vi "global_vi.vi"() -> ()   [LabVIEW 2020]
panel:
  out "A":dbl
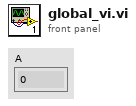
[diagram p1: front panel]
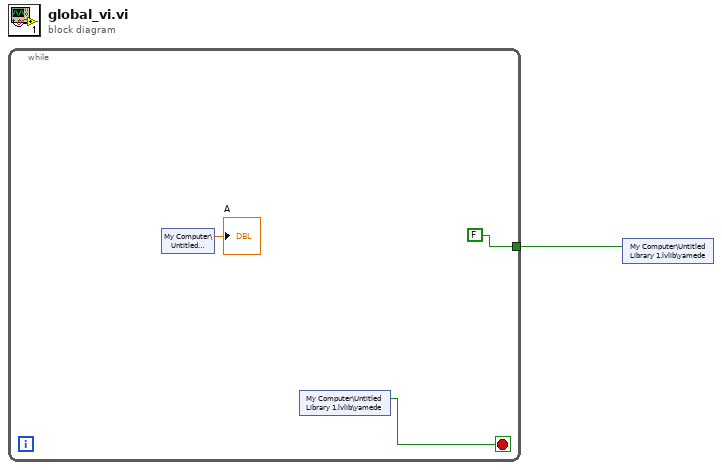
[diagram p0: block diagram]
diagram:
  n1 = while {
    tunnel: [FALSE] -> w1
    stop <- w3 stop-if-true
    n2 = shared-variable "My Computer\\Untitled Library 1.lvlib\\A"() -> (→"A":dbl)  [unwired: 1 in, 1 out]
    n3 = shared-variable "My Computer\\Untitled Library 1.lvlib\\yamede"() -> (w3:bool)  [unwired: 1 in, 1 out]
  }
  n4 = shared-variable "My Computer\\Untitled Library 1.lvlib\\yamede"(w1) -> ()  [unwired: 1 in, 1 out]
